vi "Correlated Digital Output.vi"() -> ()   [LabVIEW 2009]
doc: "I. Description:\nThis example demonstrates how to output a continuous digital pattern using an external clock.\n\nII. Instructions for Running:\n1. Select the Physical Channel to correspond to where your signal is output on the DAQ device.\n2. Select the Clock Source for the generation.\n3. Specify the Rate of the output digital pattern.\n4. Enter the digital pattern data.\n\nIII. Block Diagram Steps:\n1. Create an Digital Output Channel. \n2. Call the DAQmx (Sample Clock) VI which sets the sample clock rate. Additionally, set the sample mode to continuous.\n3. Write the data to the output buffer.\n4. Call the Start VI\n5. Loop continuously until the user presses the Stop button. Check for errors every 100 ms using the Is Task Done? VI\n6. Call the Clear Task VI to clear the Task.\n7. Use the popup dialog box to display an error or warning if any.\n\nIV. I/O Connections Overview:\nMake sure your signal output terminal matches the Physical Channel I/O Control. Also, make sure your external clock terminal matches the Clock Source Control. For further connection information, refer to your hardware reference manual."
panel:
  in  "stop":bool
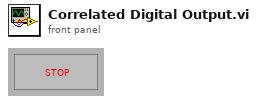
[diagram p1: front panel]
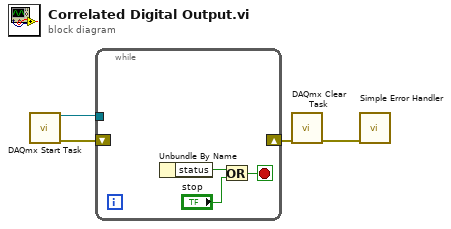
[diagram p0: block diagram]
diagram:
  n1 = call <vilib>:"DAQmx Start Task.vi"() -> ("task out"=w3:refnum<k21>, "error out"=w2:errorcluster)  [unwired: 14 in]
  n2 = while {
    tunnel: w3 -> [_]
    shift-right: [_] -> w1
    shift-left: w2 -> [_]
    stop <- w6 stop-if-true
    n3 = Unbundle By Name() -> ("status"=w5:bool)  [unwired: 1 in]
    n4 = Or(x=w5, y="stop") -> (x .or. y?=w6:bool)
  }
  n5 = call <vilib>:"DAQmx Clear Task.vi"("error in"=w1) -> ("error out"=w4:errorcluster)  [unwired: 14 in]
  n6 = call <vilib>:"Simple Error Handler.vi"("error in (no error)"=w4) -> ()  [unwired: 4 in, 5 out]
